vi "MultiplexSandbox.vi"() -> ()   [LabVIEW 2019]
uses:
  8d4a871f-ea0f-4aa7-a547-4d24cb021f7c.vi
  <vilib>/gpm_packages/@cs/event-logger/Source/Composed Log/LoggerReference/LoggerReference.lvclass
  7cb621b1-baf2-4cf0-84d6-a805fdf9e794.vi
  <vilib>/gpm_packages/@cs/Network-interface/Source/Network Messenger/Network Messenger.lvclass
  cbdfa282-940e-4c4d-bd65-94c429f3b630.vi
  <vilib>/Analysis/NI_AALBase.lvlib
  <vilib>/gpm_packages/@cs/Network-interface/Source/Network Messenger/Multiplexed Messenger/Multiplexed Messenger.lvclass
  <vilib>/Analysis/baseanly.llb/Mean (DBL).vi
  <vilib>/gpm_packages/@cs/Network-interface/Source/Network Messenger/IPacket Return/IPacket Return.lvclass
panel:
  out "error out":errorcluster
  out "Array":dbl[](array[numeric])
  out "min value":dbl
  out "max value":dbl
  out "mean":dbl format="%0.6f"
  out "Cycle Time":dbl
  out "Msg":string
  in  "String":string
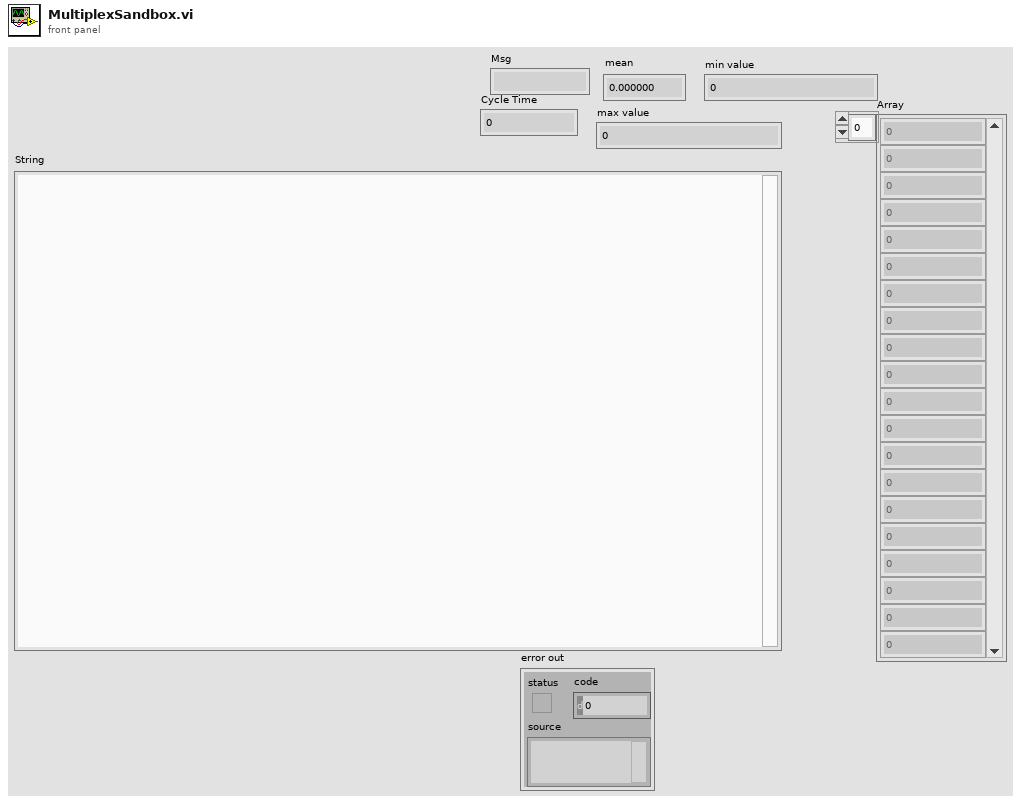
[diagram p1: front panel]
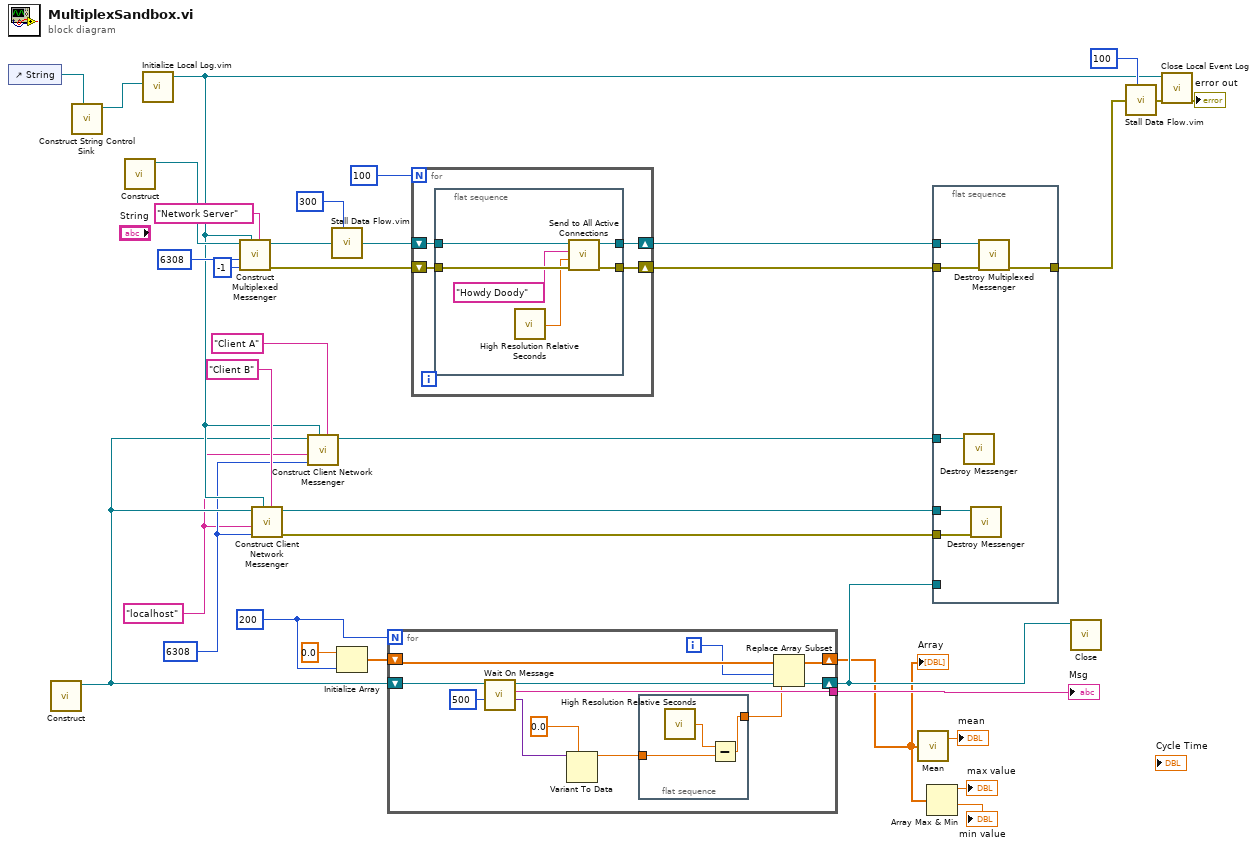
[diagram p0: block diagram]
diagram:
  w1 = 200 ("dimension size")
  w5 = u16 6308 ("Remote Port or Service Name")
  w4 = "localhost" ("Remote IP")
  n1 = control-ref of="String"() -> (w32:refnum<vi>)
  n2 = call <vilib>:"Construct.vi"() -> ("QueuePacketReturn out"=w6:refnum<class "QueuePacketReturn.lvclass">)  [unwired: 10 in, 1 out]
  n3 = call <vilib>:"Construct String Control Sink.vi"("Str Refnum"=w32) -> ("String Control Sink out"=w33:refnum<class "String Control Sink.lvclass">)  [unwired: 10 in]
  n4 = call <vilib>:"Construct.vi"() -> ("QueuePacketReturn out"=w10:refnum<class "QueuePacketReturn.lvclass">)  [unwired: 10 in, 1 out]
  n5 = call "Initialize Local Log.vim"("Startup Sink(s)"=w33) -> ("Log Instance Reference"=w7:refnum<class "LoggerReference.lvclass">)  [unwired: 8 in, 2 out]
  n6 = call <vilib>:"Construct Multiplexed Messenger.vi"("Log Alias"="Network Server", "Log Instance"=w7, "Connections To Make"=-1, "Port"=u16 6308, "Packet Return"=w10) -> ("error out"=w13:errorcluster, "Multiplexed Messenger Out"=w12:refnum<data-value>)  [unwired: 5 in]
  n7 = call <vilib>:"Construct Client Network Messenger.vi"("Log Alias"="Client B", "Log Instance"=w7, "Remote Port or Service Name"=w5, "Remote IP"=w4, "Packet Return"=w6) -> ("error out"=w26:errorcluster, "Network Node"=w27:refnum<data-value>)  [unwired: 5 in]
  n8 = call <vilib>:"Construct Client Network Messenger.vi"("Log Alias"="Client A", "Log Instance"=w7, "Remote Port or Service Name"=w5, "Remote IP"=w4, "Packet Return"=w6) -> ("Network Node"=w3:refnum<data-value>)  [unwired: 5 in, 1 out]
  n9 = call "Stall Data Flow.vim"("value in"=w12, "milliseconds to wait"=u32 300) -> ("value out"=w24:refnum<data-value>)  [unwired: 1 out]
  n10 = Initialize Array(0.0 ("element"), w1) -> (w16:dbl[])
  n11 = for {
    N: w1 -> [_]
    tunnel: [w45] -> w29
    shift-right: [w43] -> w28
    shift-left: w6 -> [w46]
    shift-right: [w39] -> w15
    shift-left: w16 -> [w38]
    i -> [w36]
    n12 = call <vilib>:"Wait On Message.vi"("timeout in ms (-1)"=500, "QueuePacketReturn in"=w46) -> ("Data"=w42:variant, "Msg"=w45:string, "QueuePacketReturn out"=w43:refnum<class "QueuePacketReturn.lvclass">)  [unwired: 5 in, 2 out]
    n13 = Variant To Data(type=0.0, Variant=w42) -> (data=w40:dbl)  [unwired: 1 in, 1 out]
    n14 = flat-sequence {
      tunnel: [w48] -> w37
      tunnel: w40 -> [w47]
      frame #0 {
        n15 = call <vilib>:"High Resolution Relative Seconds.vi"() -> ("relative seconds"=w49:dbl)
        n16 = Subtract(x=w49, y=w47) -> (x-y=w48:dbl)
      }
    }
    n17 = Replace Array Subset(array=w38, new element=w37, index=w36) -> (w39:dbl[])
  }
  "Msg" <- w29
  "Array" <- w15
  n18 = for {
    N: 100 -> [_]
    shift-right: [w51] -> w30
    shift-left: w13 -> [w52]
    shift-right: [w53] -> w31
    shift-left: w24 -> [w50]
    n19 = flat-sequence {
      tunnel: [w57] -> w53
      tunnel: w52 -> [w58]
      tunnel: [w56] -> w51
      tunnel: w50 -> [w59]
      frame #0 {
        n20 = call <vilib>:"High Resolution Relative Seconds.vi"() -> ("relative seconds"=w54:dbl)
        n21 = call <vilib>:"Send to All Active Connections.vi"("error in (no error)"=w58, "Data"=w54, "Message"="Howdy Doody", "Multiplexed Messenger In"=w59) -> ("error out"=w56:errorcluster, "Multiplexed Messenger Out"=w57:refnum<data-value>)  [unwired: 6 in]
      }
    }
  }
  n22 = call-poly <vilib>:"Mean.vi"("X"=w15) -> ("mean"=→"mean":dbl)  [unwired: 1 out]
  n23 = Array Max & Min(array=w15) -> (max value=→"max value":dbl, min value=→"min value":dbl)  [unwired: 2 out]
  n24 = flat-sequence {
    tunnel: w31 -> [w62]
    tunnel: w30 -> [w63]
    tunnel: w28 -> [_]
    tunnel: w27 -> [w65]
    tunnel: w26 -> [w64]
    tunnel: [w61] -> w25
    tunnel: w3 -> [w60]
    frame #0 {
      n25 = call <vilib>:"Destroy Messenger.vi"("Network Client Reference In"=w60) -> ()  [unwired: 10 in, 1 out]
      n26 = call <vilib>:"Destroy Messenger.vi"("error in (no error)"=w64, "Network Client Reference In"=w65) -> ()  [unwired: 9 in, 1 out]
      n27 = call <vilib>:"Destroy Multiplexed Messenger.vi"("error in (no error)"=w63, "Multiplexed Messenger In"=w62) -> ("error out"=w61:errorcluster)  [unwired: 9 in]
    }
  }
  n28 = call <vilib>:"Close.vi"("QueuePacketReturn in"=w28) -> ()  [unwired: 10 in, 1 out]
  n29 = call "Stall Data Flow.vim"("value in"=w25, "milliseconds to wait"=u32 100) -> ("value out"=w35:errorcluster)  [unwired: 1 out]
  n30 = call <vilib>:"Close Local Event Log.vi"("error in (no error)"=w35, "Log Instance"=w7) -> ("error out"=→"error out":errorcluster)  [unwired: 9 in]
